vi "FromStringCreator.vi"(4 "±í†Î”µ“þ":T1) -> (1 "表單字串":string)   [LabVIEW 2012, in "Http.lvclass"]
uses:
  Http.lvclass
  HttpData.ctl
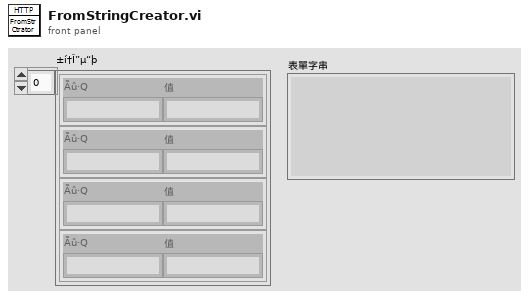
[diagram p1: front panel]
types:
  T1 = typedef "Http.lvclass/HttpData.ctl" = cluster{"Ãû·Q":string, "值":string}[]
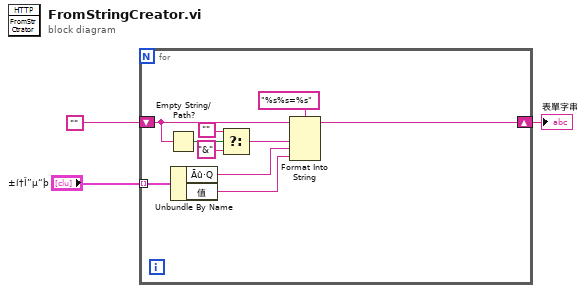
[diagram p0: block diagram]
diagram:
  n1 = for {
    tunnel: "±í†Î”µ“þ" -> [w13] mode=indexing
    shift-right: [w5] -> w1
    shift-left: "" -> [w10]
    n2 = Empty String/Path?(string/path=w10) -> (empty?=w9:bool)
    n3 = Unbundle By Name(w13) -> ("Ãû·Q"=w12:string, "值"=w11:string)
    n4 = Select(t="", s=w9, f="&") -> (s? t:f=w6:string)
    n5 = Format Into String(format string="%s%s=%s" ("格式字符串"), initial string=w10, w6, w12, w11) -> (resulting string=w5:string)  [unwired: 1 in, 1 out]
  }
  "表單字串" <- w1
